vi "DegToRadian_.vi"(5 "Angle deg":dbl format="%_10g") -> (2 "Angle radians":dbl format="%_10g")   [LabVIEW 2010]
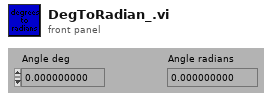
[diagram p1: front panel]
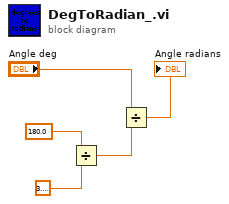
[diagram p0: block diagram]
diagram:
  n1 = Divide(x=180.0, y=3.141592653589793) -> (x/y=w2:dbl)
  n2 = Divide(x="Angle deg", y=w2) -> (x/y=→"Angle radians":dbl)
